vi "Error handler_CleanUp.vi"(5 "Error In":errorcluster) -> (19 "Error Out":errorcluster)   [LabVIEW 2019, in "Error handler.lvclass"]
uses:
  Error handler.lvclass
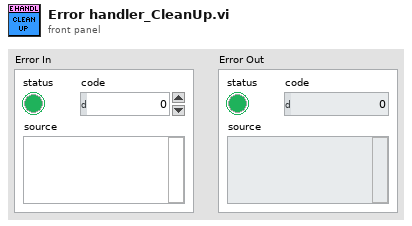
[diagram p1: front panel]
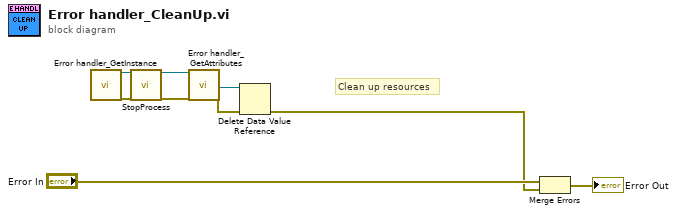
[diagram p0: block diagram]
diagram:
  # "Clean up resources"
  n1 = call "Error handler_GetInstance.vi"() -> ("reference out"=w4:refnum<class "Error handler.lvclass">, "error out"=w3:errorcluster)  [unwired: 15 in, 3 out]
  n2 = call "StopProcess.vi"("reference in"=w4, "Error In"=w3) -> ("reference out"=w1:refnum<class "Error handler.lvclass">, "Error Out"=w2:errorcluster)  [unwired: 16 in]
  n3 = call "Error handler_GetAttributes.vi"("reference in"=w1, "error in (no error)"=w2) -> ("DataRef"=w7:refnum<data-value>, "error out"=w8:errorcluster)  [unwired: 14 in, 2 out]
  n4 = Delete Data Value Reference(data value reference=w7, error in=w8) -> (error out=w5:errorcluster)  [unwired: 1 out]
  n5 = Merge Errors("Error In", w5) -> (→"Error Out":errorcluster)
